vi "Reset Graph ROI.vi"(8 "error in (no error)":errorcluster, 11 "Detail Graph. in":refnum<class "Detail Graph.lvclass">) -> (0 "error out":errorcluster, 3 "Detail Graph. out":refnum<class "Detail Graph.lvclass">)   [LabVIEW 2023, in "Detail Graph.lvclass"]
uses:
  Detail Graph.lvclass
  Detail Graph.lvclass/Detail Graph.ctl
  Base Graph/Base Graph.lvclass
  D:/git/Graph-Classes/Base Graph/Base Graph.lvclass
  D:/git/Graph-Classes/Detail Graph/Detail Graph.lvclass
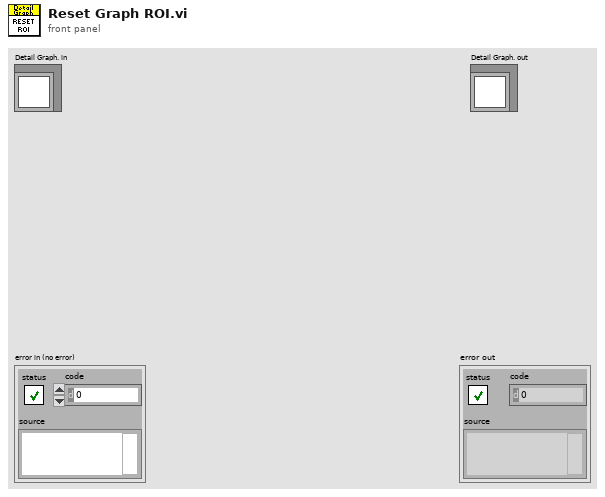
[diagram p1: front panel]
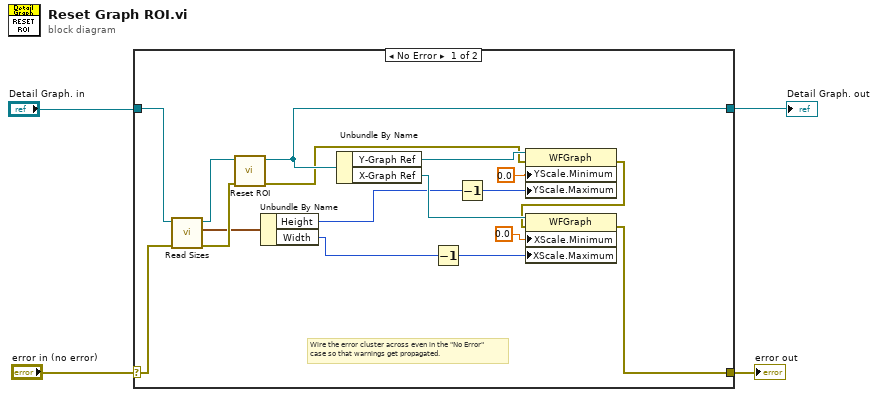
[diagram p0: block diagram]
diagram:
  n1 = case shown="No Error" "error in (no error)" {
    selector: "error in (no error)" -> [w16 w23]
    tunnel: [w5 w23] -> w3
    tunnel: [w14 w22] -> w2
    tunnel: "Detail Graph. in" -> [w17 w22]
    frame No Error {
      # "Wire the error cluster across even in the \"No Error\"\ncase so that warnings get propagated."
      n2 = call "Read Sizes.vi"("error in (no error)"=w16, "TG Base Graph in"=w17) -> ("error out"=w13:errorcluster, "Sizes"=w12:cluster{"Height":u32, "Width":u32}, "TG Base Graph out"=w15:refnum<class "Detail Graph.lvclass">)  [unwired: 7 in]
      n3 = call "Reset ROI.vi"("error in (no error)"=w13, "TG Base Graph in"=w15) -> ("error out"=w7:errorcluster, "TG Base Graph out"=w14:refnum<class "Detail Graph.lvclass">)  [unwired: 8 in]
      n4 = Unbundle By Name(w12) -> ("Height"=w11:u32, "Width"=w9:u32)
      n5 = Unbundle By Name(w14) -> ("Y-Graph Ref"=w21:refnum<vi>, "X-Graph Ref"=w20:refnum<vi>)
      n6 = Decrement(x=w9) -> (x-1=w8:u32)
      n7 = Decrement(x=w11) -> (x-1=w10:u32)
      n8 = property class="WFGraph"(reference=w21, error in=w7, "YScale.Minimum"=0.0 ("Y Scale.Range:Minimum"), "YScale.Maximum"=w10) -> (error out=w6:errorcluster)  [unwired: 1 out]
      n9 = property class="WFGraph"(reference=w20, error in=w6, "XScale.Minimum"=0.0 ("X Scale.Range:Minimum"), "XScale.Maximum"=w8) -> (error out=w5:errorcluster)  [unwired: 1 out]
    }
    frame Error {
    }
  }
  "error out" <- w3
  "Detail Graph. out" <- w2
